vi "Device.PACE6000.Find.vi"(7 "Devices in":T1, 8 "error in (no error)":errorcluster) -> (0 "error out":errorcluster, 5 "Devices out":T1)   [LabVIEW 2019]
uses:
  Devices.ctl
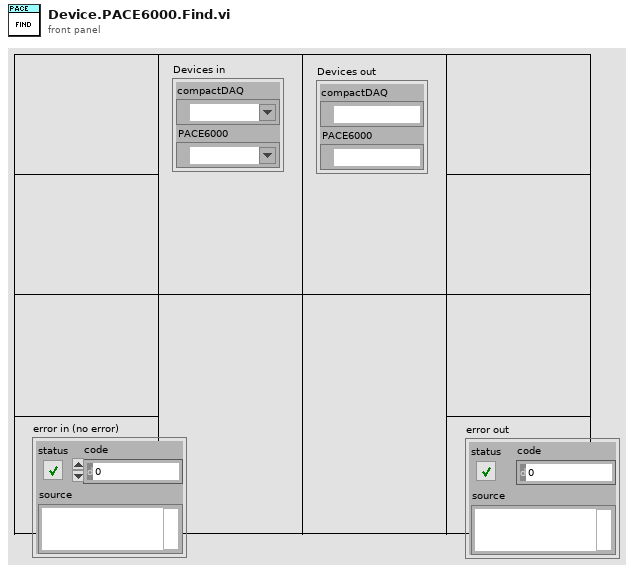
[diagram p1: front panel]
types:
  T1 = typedef "Devices.ctl" = cluster{"compactDAQ":tag, "PACE6000":refnum<visa-resource-name>}
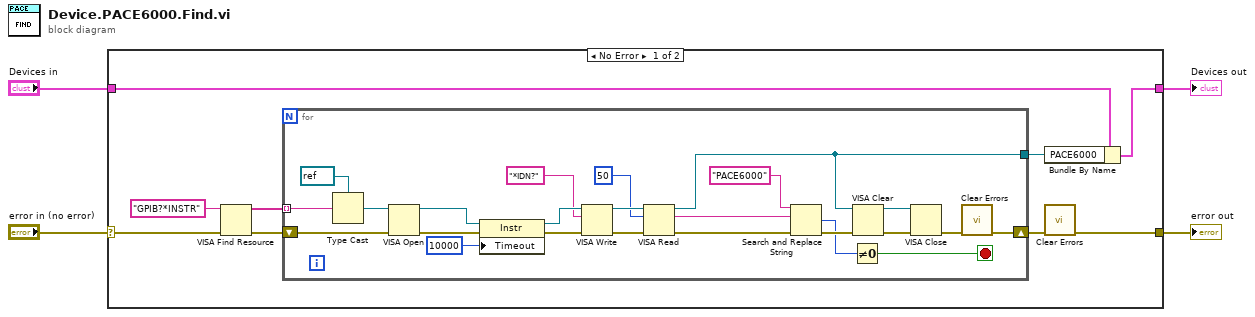
[diagram p0: block diagram]
diagram:
  n1 = case shown="No Error" "error in (no error)" {
    selector: "error in (no error)" -> [w13 w39]
    tunnel: [w5 w39] -> w2
    tunnel: "Devices in" -> [w10 w38]
    tunnel: [w8 w38] -> w4
    frame No Error {
      n2 = VISA Find Resource(8:w13, 11:"GPIB?*INSTR") -> (0:w7:errorcluster, 3:w11:string[])  [unwired: 1 in, 1 out]
      n3 = for {
        shift-right: [w14] -> w6
        shift-left: w7 -> [w36]
        tunnel: w11 -> [w37] mode=indexing
        tunnel: [w17] -> w9
        stop <- w16 stop-if-true
        n4 = Type Cast(type=refnum<visa-resource-name> refnum ("VISA resource name"), x=w37) -> (*(type *) &x=w35:refnum<visa-resource-name>)
        n5 = VISA Open(error in (no error)=w36, VISA resource name=w35) -> (VISA resource name=w32:refnum<visa-resource-name>, error out=w33:errorcluster)  [unwired: 3 in]
        n6 = property class="Instr"(reference=w32, error in=w33, "Timeout"=u32 10000 ("General Settings:Timeout Value")) -> (reference out=w29:refnum<visa-resource-name>, error out=w30:errorcluster)
        n7 = VISA Write(VISA resource name=w29, write buffer="*IDN?", error in (no error)=w30) -> (VISA resource name out=w26:refnum<visa-resource-name>, error out=w27:errorcluster)  [unwired: 1 out]
        n8 = VISA Read(VISA resource name=w26, byte count=u32 50, error in (no error)=w27) -> (VISA resource name out=w17:refnum<visa-resource-name>, read buffer=w22:string, error out=w24:errorcluster)  [unwired: 1 out]
        n9 = Search and Replace String(input string="PACE6000" ("search string"), search string=w22, error in=w24) -> (number of replacements=w18:i32, error out=w21:errorcluster)  [unwired: 5 in, 2 out]
        n10 = Not Equal To 0?(x=w18) -> (x != 0?=w16:bool)
        n11 = VISA Clear(VISA resource name=w17, error in (no error)=w21) -> (VISA resource name out=w19:refnum<visa-resource-name>, error out=w20:errorcluster)
        n12 = VISA Close(VISA resource name=w19, error in (no error)=w20) -> (error out=w15:errorcluster)
        n13 = call <vilib>:"Clear Errors.vi"("error in (no error)"=w15) -> ("error out"=w14:errorcluster)  [unwired: 5 in, 1 out]
      }
      n14 = Bundle By Name(cluster=w10, "PACE6000"=w9) -> (w8:T1)
      n15 = call <vilib>:"Clear Errors.vi"("error in (no error)"=w6) -> ("error out"=w5:errorcluster)  [unwired: 5 in, 1 out]
    }
    frame Error {
    }
  }
  "Devices out" <- w4
  "error out" <- w2
